vi "Move Node.vi"(8 "error in (no error)":errorcluster, 11 "message value":string) -> (0 "error out":errorcluster)   [LabVIEW 2013, in "Standard Editor.lvlib"]
doc: "This VI moves the nodes in the editor.\nIt cant use the default move mapping on CEF when moving on the same parent as it will delet mappings.\nIt also handles the minimun point to which you can move the node, to prevent moving tags and mappings"
uses:
  Standard Editor.lvlib
  Controls/MoveMessage.ctl
  <vilib>/NI/Configuration Framework/Node/NodeRef.ctl
  <vilib>/NI/Configuration Framework/Node/NISE_CEF_Node.lvclass
  <vilib>/NI/Configuration Framework/Node/NISE_CEF_Node.lvclass/NISE_CEF_Node.ctl
  <vilib>/NI/Configuration Framework/Node/ReadChildren.vi
  <vilib>/NI/Configuration Framework/Node/WriteChildren.vi
  <vilib>/NI/Configuration Framework/Node/ReadParent.vi
  <vilib>/NI/Configuration Framework/NISE_CEF_TreeControl.lvlib
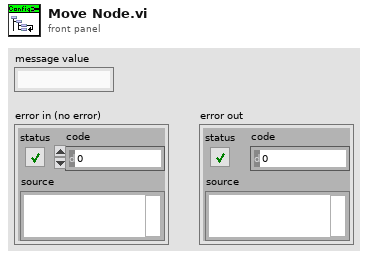
[diagram p1: front panel]
types:
  T1 = typedef "Standard Editor.lvlib/MoveMessage.ctl" = cluster{"node ref":T2, "new parent":T2, "Index":i32}
  T2 = typedef "NISE_CEF_Node.lvclass/NodeRef.ctl" = refnum<data-value>
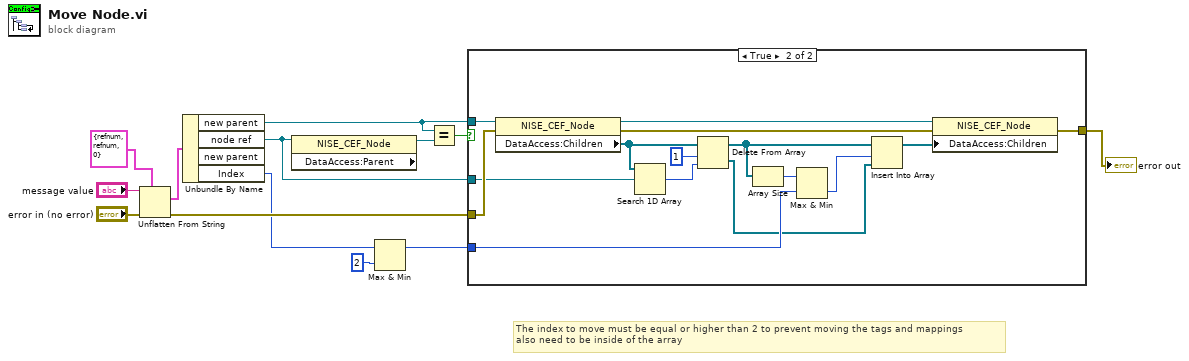
[diagram p0: block diagram]
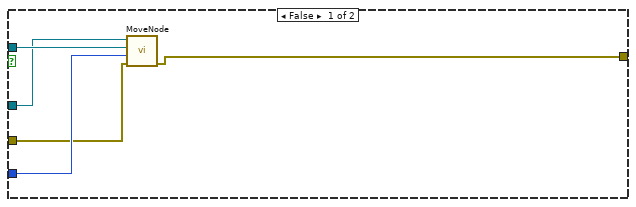
[diagram p2: hidden frame]
diagram:
  # "The index to move must be equal or higher than 2 to prevent moving the tags and mappings\nalso need to be inside of the array"
  n1 = Unflatten From String(type=T1 {"node ref"=refnum, "new parent"=refnum, "Index"=0} ("Cluster"), binary string="message value", error in (no error)="error in (no error)") -> (value=w11:T1, error out=w12:errorcluster)  [unwired: 2 in, 1 out]
  n2 = Unbundle By Name(w11) -> ("new parent"=w1:T2, "node ref"=w7:T2, "Index"=w4:i32)  [unwired: 1 out]
  n3 = property class="NISE_CEF_Node"(reference=w7) -> ("DataAccess:Parent"=w6:T2)  [unwired: 1 in, 2 out]
  n4 = Max & Min(x=w4, y=2) -> (max(x,y)=w2:i32)  [unwired: 1 out]
  n5 = Equal?(x=w1, y=w6) -> (x = y?=w5:bool)
  n6 = case shown="True" w5 {
    tunnel: w2 -> [w18 w23]
    tunnel: w1 -> [w17 w33]
    tunnel: w7 -> [w16 w28]
    tunnel: [w15 w31] -> w13
    tunnel: w12 -> [w14 w29]
    frame False {
      n7 = call <vilib>:"MoveNode.vi"("error in"=w14, "index"=w18, "new parent"=w17, "node"=w16) -> ("error out"=w15:errorcluster)  [unwired: 7 in]
    }
    frame True {
      n8 = property class="NISE_CEF_Node"(reference=w33, error in=w29) -> (reference out=w32:T2, error out=w30:errorcluster, "DataAccess:Children"=w25:T2[])
      n9 = Search 1D Array(1D array=w25, element=w28) -> (index of element=w27:i32)  [unwired: 1 in]
      n10 = Delete From Array(array=w25, length=1, index=w27) -> (deleted portion=w19:T2[], array with subset deleted=w22:T2[])
      n11 = Array Size(array=w22) -> (size(s)=w21:i32)
      n12 = Max & Min(x=w21, y=w23) -> (min(x,y)=w20:i32)  [unwired: 1 out]
      n13 = Insert Into Array(array=w22, index=w20, new element=w19) -> (w24:T2[])
      n14 = property class="NISE_CEF_Node"(reference=w32, error in=w30, "DataAccess:Children"=w24) -> (error out=w31:errorcluster)  [unwired: 1 out]
    }
  }
  "error out" <- w13
